vi "Command Lift Delay.vi"(7 "Startup":bool, 8 "Distance":dbl, 9 "Timeout":u32=5, 10 "Set Position":T1=enum."Load") -> (3 "Lift Out":dbl, 4 "Reinit":bool, 6 "Completed":bool)   [LabVIEW 2019]
uses:
  Lift/Lift Enum States.ctl
  Drive/Drive Globals.vi
  Lift/Lift Globals.vi
panel:
  in  "Lift Allowable Error Down":dbl=100.0
  out "Current Error":dbl
  in  "kP Max Down":dbl=-1.0
  in  "kP Max Up":dbl=1.0
  in  "Lift Allowable Error Up":dbl=1000.0
  in  "kP Down":dbl=4.18e-05
  in  "kP Up":dbl=0.00017
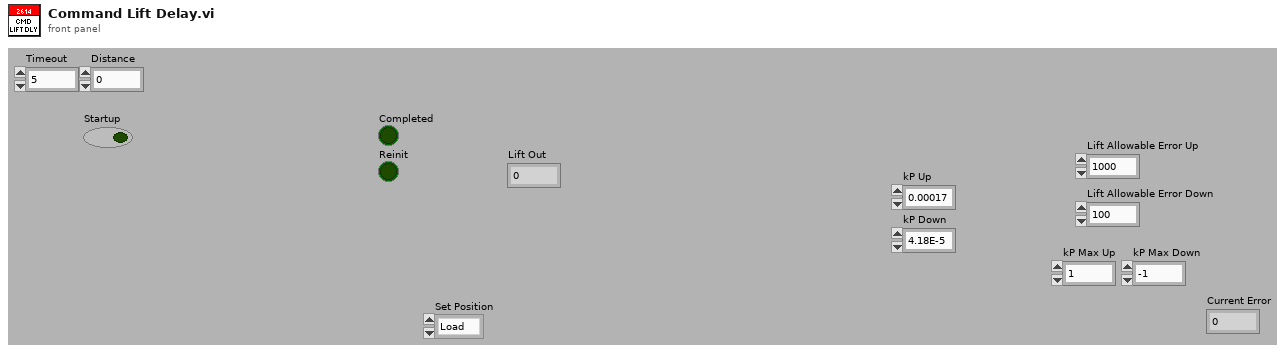
[diagram p1: front panel]
types:
  T1 = typedef "Lift Enum States.ctl" = enum16{"Climb", "Load", "Portal", "Switch", "Scale High", "Scale Mid", "Scale Low", "Exchange", "Stow", "Current Position"}
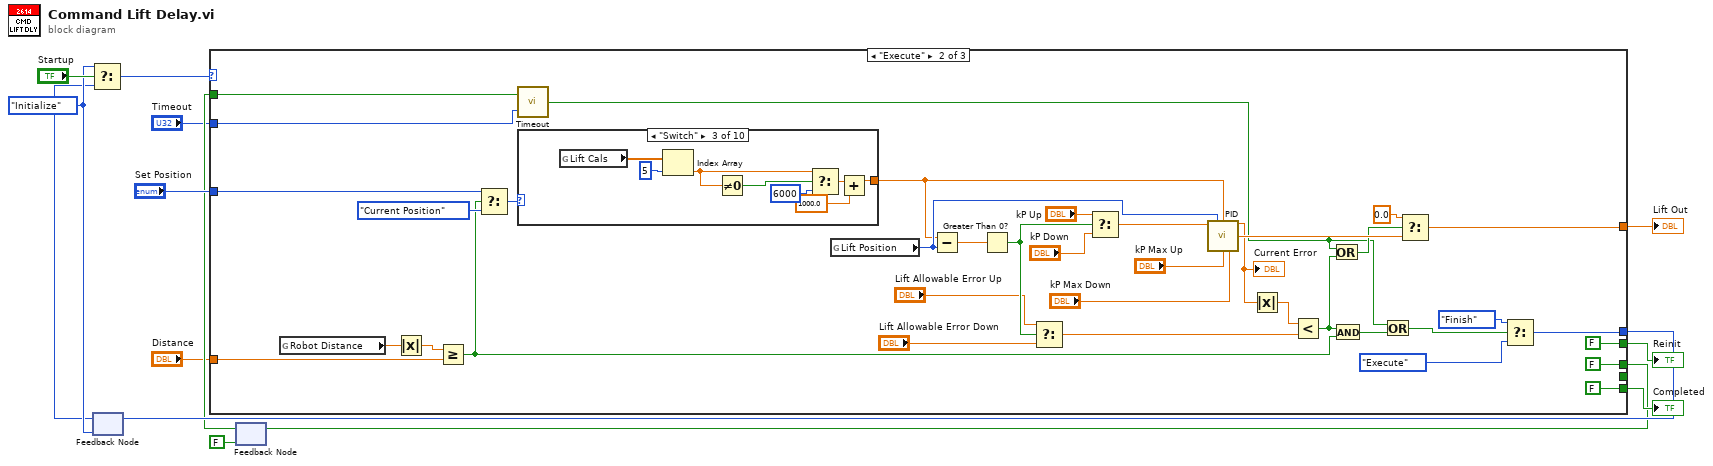
[diagram p0: block diagram]
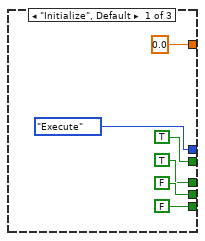
[diagram p2: hidden frame]
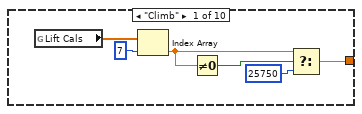
[diagram p3: hidden frame]
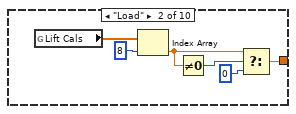
[diagram p4: hidden frame]
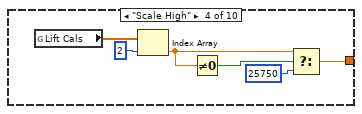
[diagram p5: hidden frame]
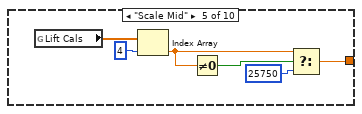
[diagram p6: hidden frame]
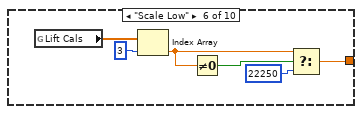
[diagram p7: hidden frame]
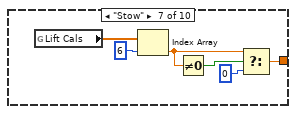
[diagram p8: hidden frame]
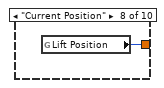
[diagram p9: hidden frame]
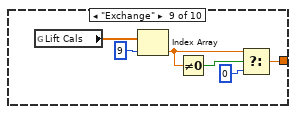
[diagram p10: hidden frame]
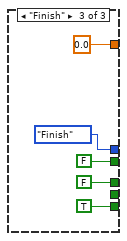
[diagram p12: hidden frame]
diagram:
  w12 = enum16{"Initialize", "Execute", "Finish"}."Initialize"
  n1 = feedback #1(w12) -> (w8:enum16{"Initialize", "Execute", "Finish"})
  n2 = Select(t=w12, s="Startup", f=w8) -> (s? t:f=w13:enum16{"Initialize", "Execute", "Finish"})
  n3 = feedback #2(FALSE) -> (w4:bool)
  n4 = case shown="\"Execute\"" w13 {
    tunnel: [FALSE FALSE TRUE] -> w11
    tunnel: [TRUE FALSE FALSE] -> w10
    tunnel: [enum16{"Initialize", "Execute", "Finish"}."Execute" w54 enum16{"Initialize", "Execute", "Finish"}."Finish"] -> w9
    tunnel: [0.0 ("Right Wheel Velocity") w27 0.0] -> w7
    tunnel: "Set Position" -> [_ w49 _]
    tunnel: [FALSE _ _] -> _
    tunnel: [TRUE FALSE FALSE] -> w5
    tunnel: w4 -> [_ w53 _]
    tunnel: "Timeout" -> [_ w52 _]
    tunnel: "Distance" -> [_ w46 _]
    frame "Initialize", Default {
    }
    frame "Execute" {
      n5 = global read "Drive Globals.vi" "Robot Distance"() -> (w48:dbl)
      n6 = Absolute Value(x=w48) -> (abs(x)=w47:dbl)
      n7 = Greater Or Equal?(x=w47, y=w46) -> (x >= y?=w43:bool)
      n8 = Select(t=w49, s=w43, f=Lift_Enum_States."Current Position") -> (s? t:f=w50:T1)
      n9 = call "Timeout.vi"("Timeout"=w52, "Initialize"=w53) -> ("Timed Out?"=w21:bool)
      n10 = case shown="\"Switch\"" w50 {
        tunnel: [w58 w65 w71 w78 w84 w90 w98 w102 w103 _] -> w25
        frame "Climb" {
          n11 = global read "Lift Globals.vi" "Lift Cals"() -> (w63:dbl[])
          n12 = Index Array(array=w63, index=7) -> (element=w60:dbl)
          n13 = Not Equal To 0?(x=w60) -> (x != 0?=w61:bool)
          n14 = Select(t=w60, s=w61, f=25750 ("Lift Position")) -> (s? t:f=w58:dbl)
        }
        frame "Load" {
          n15 = global read "Lift Globals.vi" "Lift Cals"() -> (w69:dbl[])
          n16 = Index Array(array=w69, index=8) -> (element=w66:dbl)
          n17 = Not Equal To 0?(x=w66) -> (x != 0?=w67:bool)
          n18 = Select(t=w66, s=w67, f=0 ("Lift Position")) -> (s? t:f=w65:dbl)
        }
        frame "Switch" {
          n19 = global read "Lift Globals.vi" "Lift Cals"() -> (w77:dbl[])
          n20 = Index Array(array=w77, index=5) -> (element=w73:dbl)
          n21 = Not Equal To 0?(x=w73) -> (x != 0?=w75:bool)
          n22 = Select(t=w73, s=w75, f=6000 ("Lift Position")) -> (s? t:f=w72:dbl)
          n23 = Add(x=w72, y=1000.0) -> (x+y=w71:dbl)
        }
        frame "Scale High" {
          n24 = global read "Lift Globals.vi" "Lift Cals"() -> (w83:dbl[])
          n25 = Index Array(array=w83, index=2) -> (element=w79:dbl)
          n26 = Not Equal To 0?(x=w79) -> (x != 0?=w81:bool)
          n27 = Select(t=w79, s=w81, f=25750 ("Lift Position")) -> (s? t:f=w78:dbl)
        }
        frame "Scale Mid" {
          n28 = global read "Lift Globals.vi" "Lift Cals"() -> (w89:dbl[])
          n29 = Index Array(array=w89, index=4) -> (element=w85:dbl)
          n30 = Not Equal To 0?(x=w85) -> (x != 0?=w87:bool)
          n31 = Select(t=w85, s=w87, f=25750 ("Lift Position")) -> (s? t:f=w84:dbl)
        }
        frame "Scale Low" {
          n32 = global read "Lift Globals.vi" "Lift Cals"() -> (w95:dbl[])
          n33 = Index Array(array=w95, index=3) -> (element=w91:dbl)
          n34 = Not Equal To 0?(x=w91) -> (x != 0?=w93:bool)
          n35 = Select(t=w91, s=w93, f=22250 ("Lift Position")) -> (s? t:f=w90:dbl)
        }
        frame "Stow" {
          n36 = global read "Lift Globals.vi" "Lift Cals"() -> (w101:dbl[])
          n37 = Index Array(array=w101, index=6) -> (element=w97:dbl)
          n38 = Not Equal To 0?(x=w97) -> (x != 0?=w99:bool)
          n39 = Select(t=w97, s=w99, f=0 ("Lift Position")) -> (s? t:f=w98:dbl)
        }
        frame "Current Position" {
          n40 = global read "Lift Globals.vi" "Lift Position"() -> (w102:i32)
        }
        frame "Exchange" {
          n41 = global read "Lift Globals.vi" "Lift Cals"() -> (w108:dbl[])
          n42 = Index Array(array=w108, index=9) -> (element=w104:dbl)
          n43 = Not Equal To 0?(x=w104) -> (x != 0?=w106:bool)
          n44 = Select(t=w104, s=w106, f=0 ("Lift Position")) -> (s? t:f=w103:dbl)
        }
        frame "Portal" {
        }
      }
      n45 = global read "Lift Globals.vi" "Lift Position"() -> (w35:i32)
      n46 = Subtract(x=w25, y=w35) -> (x-y=w36:dbl)
      n47 = Greater Than 0?(x=w36) -> (x > 0?=w31:bool)
      n48 = Select(t="Lift Allowable Error Up", s=w31, f="Lift Allowable Error Down") -> (s? t:f=w30:dbl)
      n49 = Select(t="kP Up", s=w31, f="kP Down") -> (s? t:f=w39:dbl)
      n50 = call "PID.vi"("Kp"=w39, "Process Variable"=w35, "Goal"=w25, "Max Ouput"="kP Max Up", "Min Output"="kP Max Down") -> ("Current Error"=w32:dbl, "Command"=w41:dbl)  [unwired: 8 in, 1 out]
      "Current Error" <- w32
      n51 = Absolute Value(x=w32) -> (abs(x)=w40:dbl)
      n52 = Less?(x=w40, y=w30) -> (x < y?=w22:bool)
      n53 = Or(x=w21, y=w22) -> (x .or. y?=w26:bool)
      n54 = And(x=w22, y=w43) -> (x .and. y?=w23:bool)
      n55 = Or(x=w21, y=w23) -> (x .or. y?=w24:bool)
      n56 = Select(t=0.0, s=w26, f=w41) -> (s? t:f=w27:dbl)
      n57 = Select(t=enum16{"Initialize", "Execute", "Finish"}."Finish", s=w24, f=enum16{"Initialize", "Execute", "Finish"}."Execute") -> (s? t:f=w54:enum16{"Initialize", "Execute", "Finish"})
    }
    frame "Finish" {
    }
  }
  "Completed" <- w11
  "Reinit" <- w10
  "Lift Out" <- w7
  n58 = feedback-in #1(w9) -> ()
  n59 = feedback-in #2(w5) -> ()
